vi "IP Configure.vi"() -> (3 "IP Configer":T1)   [LabVIEW 2017]
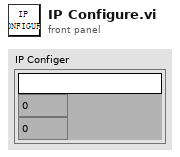
[diagram p1: front panel]
types:
  T1 = cluster{"IP_Address":string, "Port":u16, "Out Time":i32}
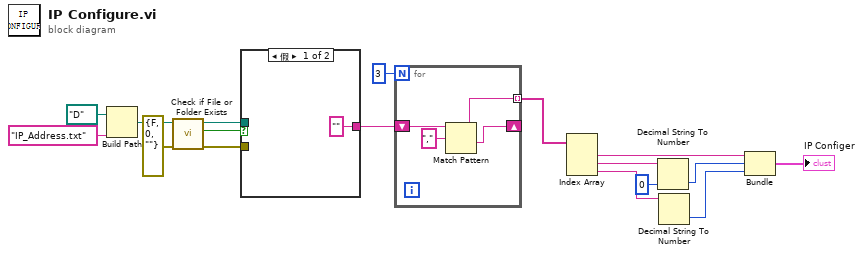
[diagram p0: block diagram]
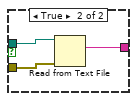
[diagram p2: hidden frame]
diagram:
  n1 = Build Path(base path=path "D:/" ("基路径"), name or relative path="IP_Address.txt" ("名称或相对路径")) -> (appended path=w15:path)
  n2 = call <vilib>:"Check if File or Folder Exists.vi"("error in (no error)"=errorcluster {"status"=FALSE, "code"=0, "source"=""}, "path"=w15) -> ("error out"=w11:errorcluster, "file or folder exists?"=w13:bool, "dup path"=w12:path)  [unwired: 7 in]
  n3 = case shown="假" w13 {
    tunnel: w12 -> [_ w21]
    tunnel: w11 -> [_ w20]
    tunnel: ["" w19] -> w10
    frame False {
    }
    frame True {
      n4 = Read from Text File(file (use dialog)=w21, error in=w20) -> (text=w19:string)  [unwired: 2 in, 3 out]
    }
  }
  n5 = for {
    N: 3 -> [_]
    shift-right: [w24] -> _
    shift-left: w10 -> [w25]
    tunnel: [w22] -> w8 mode=indexing
    n6 = Match Pattern(string=w25, regular expression="," ("正则表达式")) -> (before substring=w22:string, after substring=w24:string)  [unwired: 1 in, 2 out]
  }
  n7 = Index Array(array=w8) -> (element #1=w7:string, element #2=w6:string, element #3=w4:string)  [unwired: 3 in]
  n8 = Decimal String To Number(string=w6, default (0L)=u16 0 ("默认(0 I32)")) -> (number=w5:u16)  [unwired: 1 in, 1 out]
  n9 = Decimal String To Number(string=w4) -> (number=w3:i32)  [unwired: 2 in, 1 out]
  n10 = Bundle(w7, w5, w3) -> (→"IP Configer":cluster{string, u16, i32})  [unwired: 1 in]
